vi "2020_day03.vi"() -> ()   [LabVIEW 2021]
panel:
  out "Number of Trees (Task 2)":u64
  out "Number of Trees (Task 1)":i32
  in  "Live/Test Data Src":bool
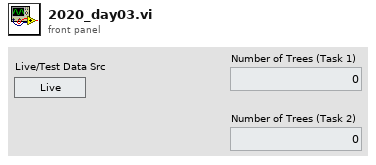
[diagram p1: front panel]
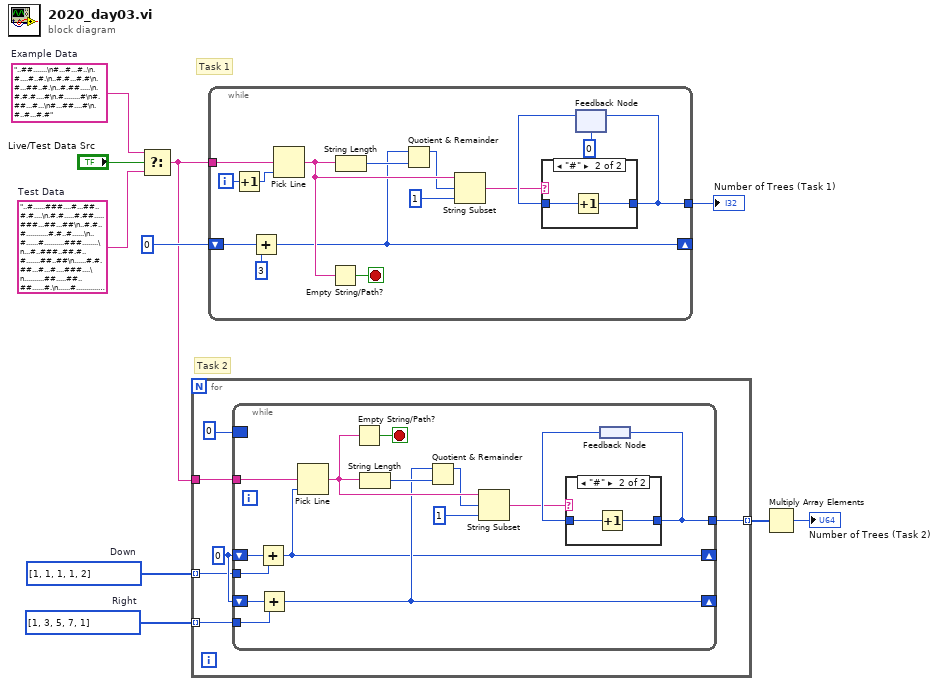
[diagram p0: block diagram]
diagram:
  w4 = i32[] [1, 3, 5, 7, 1]  # Right
  w3 = i32[] [1, 1, 1, 1, 2]  # Down
  w9 = "..#......###....#...##..#.#....\n.#.#.....#.##.....###...##...##\n..#.#..#...........#.#..#......\n..#......#..........###........\n...#..###..##.#..#.......##..##\n......#.#.##...#...#....###....\n..........##.....##..##......#.\n......#...........#............\n#....#..........#..............\n.#........##.............###.##\n....#.........#.......#.#....##\n#.#..#..#..#.......#...#....##.\n.#........#......#.##.......#..\n..#.....#####.....#....#..#..##\n.......#..##.......#......#.###\n..#.#...#......#.##...#........\n##...................#...##..#.\n......#...#.##...##.#......#..#\n.#.................#..##...#...\n...#.....#.......##.....#.#....\n.......#.#......#.....#..#..##.\n..........#........#...........\n..#.#..........................\n.#.##..#.#...#...#.........#...\n.....#....#.....#..#.....#.....\n...#.#.#.....#.#..#.......#..#.\n.....#...###...##...#......##..\n#.###......#.#...#.#.#..###....\n#.....#..##......#..........#.#\n#...............#........#.#..#\n.....#..#.........#......##.#..\n.....#.##.##..#..##............\n...#......##...............#.#.\n.#..#.#............##.#........\n#.....#..###.............##.#..\n...##..#.#..#...........#..#...\n#....#.........#.#.............\n##.#.........#..###......#.#..#\n...#...#......#.#.#.##..#.##...\n.....##............#.##.##..#..\n....#................#.##..#..#\n...#..#.......#...#..#........#\n....#...#...#................#.\n....##...............#.#...#...\n.#.....###...#.......#.##......\n....######.#..............###.#\n.#..#.........##...............\n................##.#..#....###.\n.......#............#.#..#..#..\n......#.#...............##.#...\n...#..####.#...#..#..#......#..\n....#.#...#.....#.........#..##\n.##..#...#......##....##.#.#...\n.##.#.........##...#....#......\n..#.#..#...#.#..#.......#...#.#\n.........#..#.....##..#........\n..#......#..##.....#..#...###..\n..#...#....#.#..#..#.#.#..#.#..\n...#..#####.....#......#.......\n#.#............#......#..#...#.\n.........#..........###.......#\n......#....#..#.##.#......#..#.\n...........##.#....#.#..#......\n..#...................#..#.#...\n#....##.............##....#...#\n##..#....#.........#..........#\n....#.#.#...#..#........#.##..#\n...............#...#..##..#....\n.##.......#.......#...........#\n#.........................##...\n#........#.#..#..##..####.#....\n...................##.....###..\n.#.......#..#......#......#...#\n..#.........#...#..........#...\n..........#......#....#........\n.#......#..#...#..#...##....##.\n...#.#..#..#......#.....##.####\n.......#.#....#.......#........\n#...#.#...##..##.#......#......\n.#.........#...................\n...#..........#.#......#.......\n...#.....##....#..........#....\n.#..........##..#..#..##....#.#\n.##.#..........#...#.##.......#\n#...###....#..#.#...#..#.......\n..................##...........\n..#...##.#...........#....#.##.\n..#......#..##..#....##..#...#.\n..#....#.....#.##..#.......#..#\n#...#....#..#.#....#......##...\n.......##..#..........#........\n..#.............##.#.....#...#.\n...............#....#...#...##.\n##...........#.......#.##......\n#..#...........#.........#.....\n....###.............###.##..##.\n.........#.#.....###.......#...\n..#.##....#.#..........#....#..\n#........#....##...#..#........\n......#..........###..#.#......\n.....#.#......##.....#..##...#.\n.#.......#......#...#...#...#.#\n.#..........##.......#.....##.#\n###.#...#....#.....#...#......#\n..#.#.#..#.##.#..#.............\n.....#.........................\n.#..###..#...#...#..#..#...#.#.\n#................##...##.##....\n......#...#...#..........#...#.\n..........#.....##.............\n..#.#......#........#.......#..\n........##.............#.......\n.......#......#.##.#..#........\n#.#.#....#........#..........#.\n##..##......#..#..#.....#.#..##\n##..#..........#...............\n#.....##...#.#......#.......#.#\n#.....#...#....#..#.....##.....\n##..........#.#.....#....#...##\n..##.###..#.....#.......#...#..\n.#.#.......#......###........#.\n.#..............#.#..###.......\n.#....#..##.........#..#.#.....\n....#....#.#....#..#.......##.#\n#.......#.......#.........#....\n...#....#....#.....##..#..#.#.#\n........#....#...........#.....\n.#......##.#.#.##..............\n#..#.#.....##........#........#\n##...#.#.......##.......#...#..\n#...#.....#.##...##.#.....#....\n....#..##...#........#.#...#...\n...#....#.#.#..###...##.#.....#\n......#..#.....#..#........##..\n.......#.....#.#.........#.#..#\n..#.......#.#.#.#.#....#.##...#\n.#...#........#..##..#......#..\n.#..#............#...#..#.#....\n...##......#......#............\n..#...#.#.....#.....#..##.#....\n.#......#.#......#..#.#........\n..#..........##...#.#.....#..#.\n#...#.....#..#...#.............\n..##.................#....#....\n.#....#.......#..##....#......#\n.#....###............##....##.#\n##..#........#..#...#.......#..\n.....#.....#.#.#.##.........#..\n.......#..#....#...#...#.......\n...#...#...#.#.#..#.#.....#....\n#.#........#..#.##..#..###.....\n..................#..#.........\n#.#.....#..##.........#.......#\n###..#.......#..............#..\n......#..#.....###..........#..\n....#.#...#..#...........#.#...\n...#.....#.......#.....#.#.....\n#.....##..#......##...........#\n#...###...........##..#...#.##.\n......##.##.#...#..#....#......\n...#.#......##.#......##....#.#\n..............#.#.###.......#..\n........#....#.......##..#..###\n...#.....##.#....#......##..#.#\n..##........#.....#.#..#...#...\n.#..#.##.........#.....#...#..#\n..#..#....#...........#........\n.#...#....................#....\n##.....##....#.............#.#.\n....#.#..#.#..#.#.#..........##\n.............##.#.....#..#..#..\n.#....#.....##...#.###.........\n..#........#........#.#..###...\n.##....#...#...#.......#...#.#.\n..#...#...#..##........#..#....\n..##.#..#..#.....#......#.#..#.\n.#........#..#....#..#.........\n..#.#.....#.##..#........###.#.\n.....#.##.....##.#.............\n#.........#.......#...##...#...\n..#.##.#..#..#............#....\n.##....#..#............#.....#.\n###........##.....##.#...#.....\n#......##..##.#.#.#.#.#.#..##..\n.....###.....#....#......#....#\n........#.........##...#....#.#\n.#.#.....#.#..#..##......#...#.\n...#.##....#..#.###..#..##.....\n....#..........##..#..#..#..#..\n...#..#.##..#..#....#.........#\n.....#..###.#.....#.....#..#...\n......#...#....#.##...#.#......\n.#.###..##.....##.##......##...\n.....#.#...........#.#.........\n#........#...#..#......##.#....\n..#.......##....##....#.##.#..#\n...###.#.........#......#.....#\n..#.##..#....#.....##...#.##...\n....##.##.............#...#....\n##..#...#..#..#..#.............\n.....#.....#.....#.............\n...#.##.......#..#.#.....#....#\n#.....##.........#......##.....\n.....##..........#..#...#..#...\n#...###....#.......#...##......\n.#....#..#......#.....#...#.#..\n#........#.#.#...#.....###.#.##\n##...#...##..#..#....#.........\n....#............#..#.....#....\n#......#.........##....#.......\n.#..#..#........#.............#\n.##..........#......#.......#..\n#............#..#....#.........\n....#.#.....#.##...#.....#.#...\n...#.#..#...##..#...#.#.#......\n#....#..#.........##..#.#.#..##\n.#...#..............#.......#..\n#...#.....#.#........##......##\n...#....##.####.#.........#.#.#\n....###.#..#............#.#..#.\n....#......#...#......##.#.#.#.\n.....#..#.#.##.#...##..........\n##..#...#.#...###.............#\n....#...#..#.....#.#..#..#..#..\n#..........####......#.....###.\n.........#........#.##.#...#...\n.........#..........#.#..###...\n.....##........##.........#...#\n..##....#...#.......##.........\n.....#.#......##....#...#...#..\n.##..#..##.....................\n.......#...#..#..#...##....#...\n.#...#.......###...#..#..#.....\n.......#.....##.##.#.......#..#\n.##......#...#....#..#......##.\n.##....#..#....#...#...#.......\n.........##..#..#.#.#.....##...\n...#..............#..#.....####\n.#.#.#..#.......#.......#......\n..#.#......#..........#........\n.#...#.#..#.......#..#..#..#...\n.......##.#...#..#....#.....#..\n.##...##....##...#........####.\n....#.#..##....#...#....#.#....\n.....#.....#..#..#.#.##..#.....\n..#....#..............#....#...\n..#.#.#.....##.#.....#..##.....\n....#.....#....#...#...#..#.#..\n#...#...........#..#..#........\n...#.#..#.........##.#...#..##.\n......#.#.........#.#...#......\n......#..##.###......##.#....#.\n.....#...#..#.......#..........\n.#...#.......#.....###......#..\n...........##.....#..#..#....#.\n..#....#..#...#......#.......#.\n..#...#...#.#..#....#...#......\n.......#....###.####...###.#...\n#.##.#.......#.......#....#.#.#\n.##..........#.....#..###......\n.....#...........#.##..#....#..\n........##.....#.#........##...\n#..#..#..................##....\n#...###..........#.............\n.......#.#.......#.#.......##..\n.....#.#...#....#...####.....#.\n..##.....##.......#....#.......\n##..........#...#..##....##....\n..........#..#......#........#.\n##..#....#..#....#.....##....#.\n##.##.....#...##.##.......#....\n..#..#.###.#..##.#..#..#...#...\n.#..#.....#........#...##.#....\n..#..#.....#.#......##.#.#.....\n.#..##...#.#....#...#...#.#.##.\n.........#...#....###.#.....#..\n...........###.#.#..#..#...#.#.\n##...#......##...........#..#..\n.........##..#...#.......#.....\n#......#.#..........#..#.......\n...#.................#....#....\n#....#......................##.\n##.......#..#......#.#...###.#.\n..#....#..#.#......#...........\n...#...........###.#.#.........\n..#..##.....#.....##...##......\n..#..#.#.#.#..#..#..##....#...#\n#......##.....##..##.##...#....\n#.....#.....#.#........#.......\n.#.....#.................#....#\n.###....#...#............#.#.#.\n.#...#.#......#.#..............\n....#...#......#.....#.......#.\n........#.....#..........#....#\n#..#......#...#...#.........#..\n#....#......#...##.#...#...#...\n#...#....#....#..#..#.....#..#.\n#......##..#..#.#.#..#.#.......\n..#..#...............#...##...#\n............#..............#.##\n.#.#.#......##.......#.......#.\n....#.........##.......#...###.\n.......#.#...#.#.#.......#.....\n....#..#..#...#....#.##.#.##...\n...##.##.#...#......#..........\n#.....#...#.#...#.##..##.#.....\n.......#.....#...#.#...##.#....\n.#.............#.....#....##..#\n##......#.......#...#....#.....\n.###......#.................#..\n#.#......##.........##..#......\n...#....#..........#.#.........\n..##..#.........#..............\n.....#...#..................#.#\n.............#.........#...#..#\n....#....#......#.#.......#...#\n#..#............#.#.......#...#\n..#.....#............#.........\n.#.....................###....#\n........#.####.........#.#.#...\n#...........##...#.........#..#\n...........#..#......#...#.#...\n....##...##.....#.....#........"  # Test Data
  w10 = "..##.......\n#...#...#..\n.#....#..#.\n..#.#...#.#\n.#...##..#.\n..#.##.....\n.#.#.#....#\n.#........#\n#.##...#...\n#...##....#\n.#..#...#.#"  # Example Data
  # "Task 1"
  # "Task 2"
  n1 = Select(t=w10, s="Live/Test Data Src", f=w9) -> (s? t:f=w5:string)
  n2 = for {
    tunnel: w5 -> [w15]
    tunnel: w4 -> [w13] mode=indexing
    tunnel: [w16] -> w1 mode=indexing
    tunnel: w3 -> [w12] mode=indexing
    w14 = 0 ("y")
    n3 = while {
      tunnel: w15 -> [w30]
      shift-right: [w26] -> _
      shift-left: w14 -> [w29]
      tunnel: [w23] -> w16
      shift-right: [w19] -> _
      shift-left: w14 -> [w21]
      tunnel: w12 -> [w20]
      tunnel: w13 -> [w18]
      border: u64 0 -> [_]
      stop <- w31 stop-if-true
      n4 = Add(x=w21, y=w20) -> (x+y=w19:i32)
      n5 = Add(x=w29, y=w18) -> (x+y=w26:i32)
      n6 = Pick Line(multi-line string=w30, line index=w19) -> (output string=w27:string)  [unwired: 1 in]
      n7 = Empty String/Path?(string/path=w27) -> (empty?=w31:bool)
      n8 = String Length(string=w27) -> (length=w28:i32)
      n9 = Quotient & Remainder(x=w26, y=w28) -> (x-y*floor(x/y)=w22:i32)  [unwired: 1 out]
      n10 = String Subset(string=w27, offset (0)=w22, length (rest)=1 ("length (rest)")) -> (substring=w17:string)
      n11 = feedback #1() -> (w24:u64)
      n12 = case shown="\"#\"" w17 {
        tunnel: w24 -> [w32 w34]
        tunnel: [w32 w33] -> w23
        frame Default {
        }
        frame "#" {
          n13 = Increment(x=w34) -> (x+1=w33:u64)
        }
      }
      n14 = feedback-in #1(w23) -> ()
    }
  }
  n15 = while {
    tunnel: w5 -> [w48]
    shift-right: [w41] -> _
    shift-left: 0 -> [w46]
    tunnel: [w37] -> w6
    i -> [w47]
    stop <- w49 stop-if-true
    n16 = Increment(x=w47) -> (x+1=w43:i32)
    n17 = Add(x=w46, y=3) -> (x+y=w41:i32)
    n18 = Pick Line(multi-line string=w48, line index=w43) -> (output string=w42:string)  [unwired: 1 in]
    n19 = Empty String/Path?(string/path=w42) -> (empty?=w49:bool)
    n20 = String Length(string=w42) -> (length=w44:i32)
    n21 = Quotient & Remainder(x=w41, y=w44) -> (x-y*floor(x/y)=w36:i32)  [unwired: 1 out]
    n22 = String Subset(string=w42, offset (0)=w36, length (rest)=1 ("length (rest)")) -> (substring=w35:string)
    n23 = feedback #2(0) -> (w39:i32)
    n24 = case shown="\"#\"" w35 {
      tunnel: w39 -> [w50 w52]
      tunnel: [w50 w51] -> w37
      frame Default {
      }
      frame "#" {
        n25 = Increment(x=w52) -> (x+1=w51:i32)
      }
    }
    n26 = feedback-in #2(w37) -> ()
  }
  "Number of Trees (Task 1)" <- w6
  n27 = Multiply Array Elements(1:w1) -> (0:→"Number of Trees (Task 2)":u64)
